vi "SERIAL_DecodeASCIIPacket.vi"(8 "error in":errorcluster, 9 "PacketType":string, 10 "Buffer":string, 11 "navX DevRef":T1={"SerialPortRef"={"DevStatus"={"status"=FALSE, "code"=0, "source"=""}, "Serial Port Name"=""}, "Board Information"={"WhoAmI (50 | 0x32)"=0, "Board Revision"=0, "Firmware Major Version"=0, "Firmware Minor Version"=0, "NAVX_BOARD_CAPABILITY"={"OMNIMOUNT"=FALSE, "YAW_RESET"=FALSE, "VEL_AND_DISP"=FALSE}, "NAVX_BOARD_YAW_AXIS"={"BOARD_YAW_AXIS_UP"=FALSE, "BOARD_YAW_AXIS"=0}}, "Status"={"Update Rate Hz"=0, "Accelerometer Full-Scale Range"=0, "Gyro Full-Scale Range"=0, "NAVX_OP_STATUS"=0, "NAVX_CAL_STATUS"=0, "NAVX_SELFTEST_STATUS"=0, "NAVX_SENSOR_STATUS"={"MOVING"=FALSE, "YAW_STABLE"=FALSE, "MAG_DISTURBANCE"=FALSE, "ALTITUDE_VALID"=FALSE, "SEALEVEL_PRESS_SET"=FALSE, "FUSED_HEADING_VALID"=FALSE}}, "Offsets"={"Yaw"=0.0, "Quat W"=0.0, "Quat X"=0.0, "Quat Y"=0.0, "Quat Z"=0.0}, "Update Rate (4Hz-60Hz)"=50, "Nav6Mode (YPR)"=enum."YPR", "refnum name"="", "error"={"status"=FALSE, "code"=0, "source"=""}, "Loop VI Refnum"=refnum, "Serial Port"=enum."Onboard RS-232"} {"Status"."NAVX_OP_STATUS" items=["INITIALIZING", "SELFTEST_IN_PROGRESS", "ERROR", "IMU_AUTOCAL_IN_PROGRESS", "NORMAL"]; "Status"."NAVX_CAL_STATUS" items=["IMU_CAL_STATE_MASK"=3, "IMU_CAL_INPROGRESS"=0, "IMU_CAL_ACCUMULATE"=1, "IMU_CAL_COMPLETE"=2, "MAG_CAL_COMPLETE"=4, "BARO_CAL_COMPLETE"=8]}) -> (0 "error out":errorcluster, 2 "Valid":bool, 3 "navX DevRef":T1={"SerialPortRef"={"DevStatus"={"status"=FALSE, "code"=0, "source"=""}, "Serial Port Name"=""}, "Board Information"={"WhoAmI (50 | 0x32)"=0, "Board Revision"=0, "Firmware Major Version"=0, "Firmware Minor Version"=0, "NAVX_BOARD_CAPABILITY"={"OMNIMOUNT"=FALSE, "YAW_RESET"=FALSE, "VEL_AND_DISP"=FALSE}, "NAVX_BOARD_YAW_AXIS"={"BOARD_YAW_AXIS_UP"=FALSE, "BOARD_YAW_AXIS"=0}}, "Status"={"Update Rate Hz"=0, "Accelerometer Full-Scale Range"=0, "Gyro Full-Scale Range"=0, "NAVX_OP_STATUS"=0, "NAVX_CAL_STATUS"=0, "NAVX_SELFTEST_STATUS"=0, "NAVX_SENSOR_STATUS"={"MOVING"=FALSE, "YAW_STABLE"=FALSE, "MAG_DISTURBANCE"=FALSE, "ALTITUDE_VALID"=FALSE, "SEALEVEL_PRESS_SET"=FALSE, "FUSED_HEADING_VALID"=FALSE}}, "Offsets"={"Yaw"=0.0, "Quat W"=0.0, "Quat X"=0.0, "Quat Y"=0.0, "Quat Z"=0.0}, "Update Rate (4Hz-60Hz)"=50, "Nav6Mode (YPR)"=enum."YPR", "refnum name"="", "error"={"status"=FALSE, "code"=0, "source"=""}, "Loop VI Refnum"=refnum, "Serial Port"=enum."Onboard RS-232"} {"Status"."NAVX_OP_STATUS" items=["INITIALIZING", "SELFTEST_IN_PROGRESS", "ERROR", "IMU_AUTOCAL_IN_PROGRESS", "NORMAL"]; "Status"."NAVX_CAL_STATUS" items=["IMU_CAL_STATE_MASK"=3, "IMU_CAL_INPROGRESS"=0, "IMU_CAL_ACCUMULATE"=1, "IMU_CAL_COMPLETE"=2, "MAG_CAL_COMPLETE"=4, "BARO_CAL_COMPLETE"=8]})   [LabVIEW 2014, in "navX-MXP IMU.lvlib"]
uses:
  navX-MXP IMU.lvlib
  navX Serial DevRef.ctl
  <vilib>/Rock Robotics/WPI/SerialPort/WPI_SerialPortRef.ctl
  COMMON/TypeDefs/Data TypeDefs/navX Board Information.ctl
  COMMON/TypeDefs/Value TypeDefs/navX NAVX_BOARD_CAPABILITY.ctl
  COMMON/TypeDefs/Value TypeDefs/navX NAVX_BOARD_YAW_AXIS.ctl
  COMMON/TypeDefs/Data TypeDefs/navX Status Data.ctl
  COMMON/TypeDefs/Value TypeDefs/navX NAVX_OP_STATUS.ctl
  COMMON/TypeDefs/Value TypeDefs/navX NAVX_CAL_STATUS.ctl
  COMMON/TypeDefs/Value TypeDefs/navX NAVX_SENSOR_STATUS.ctl
  TypeDefs/navX Serial Mode.ctl
  IO/NI WPI/WPI_SerialPort_USB.ctl
  COMMON/TypeDefs/Data TypeDefs/navX Vector Data.ctl
  TypeDefs/navX Raw Data.ctl
  COMMON/TypeDefs/Data TypeDefs/navX YPRH Data.ctl
  <vilib>/Rock Robotics/SystemInterfaces/Utilities/FPGA_UtilitiesRead LocalTime.vi
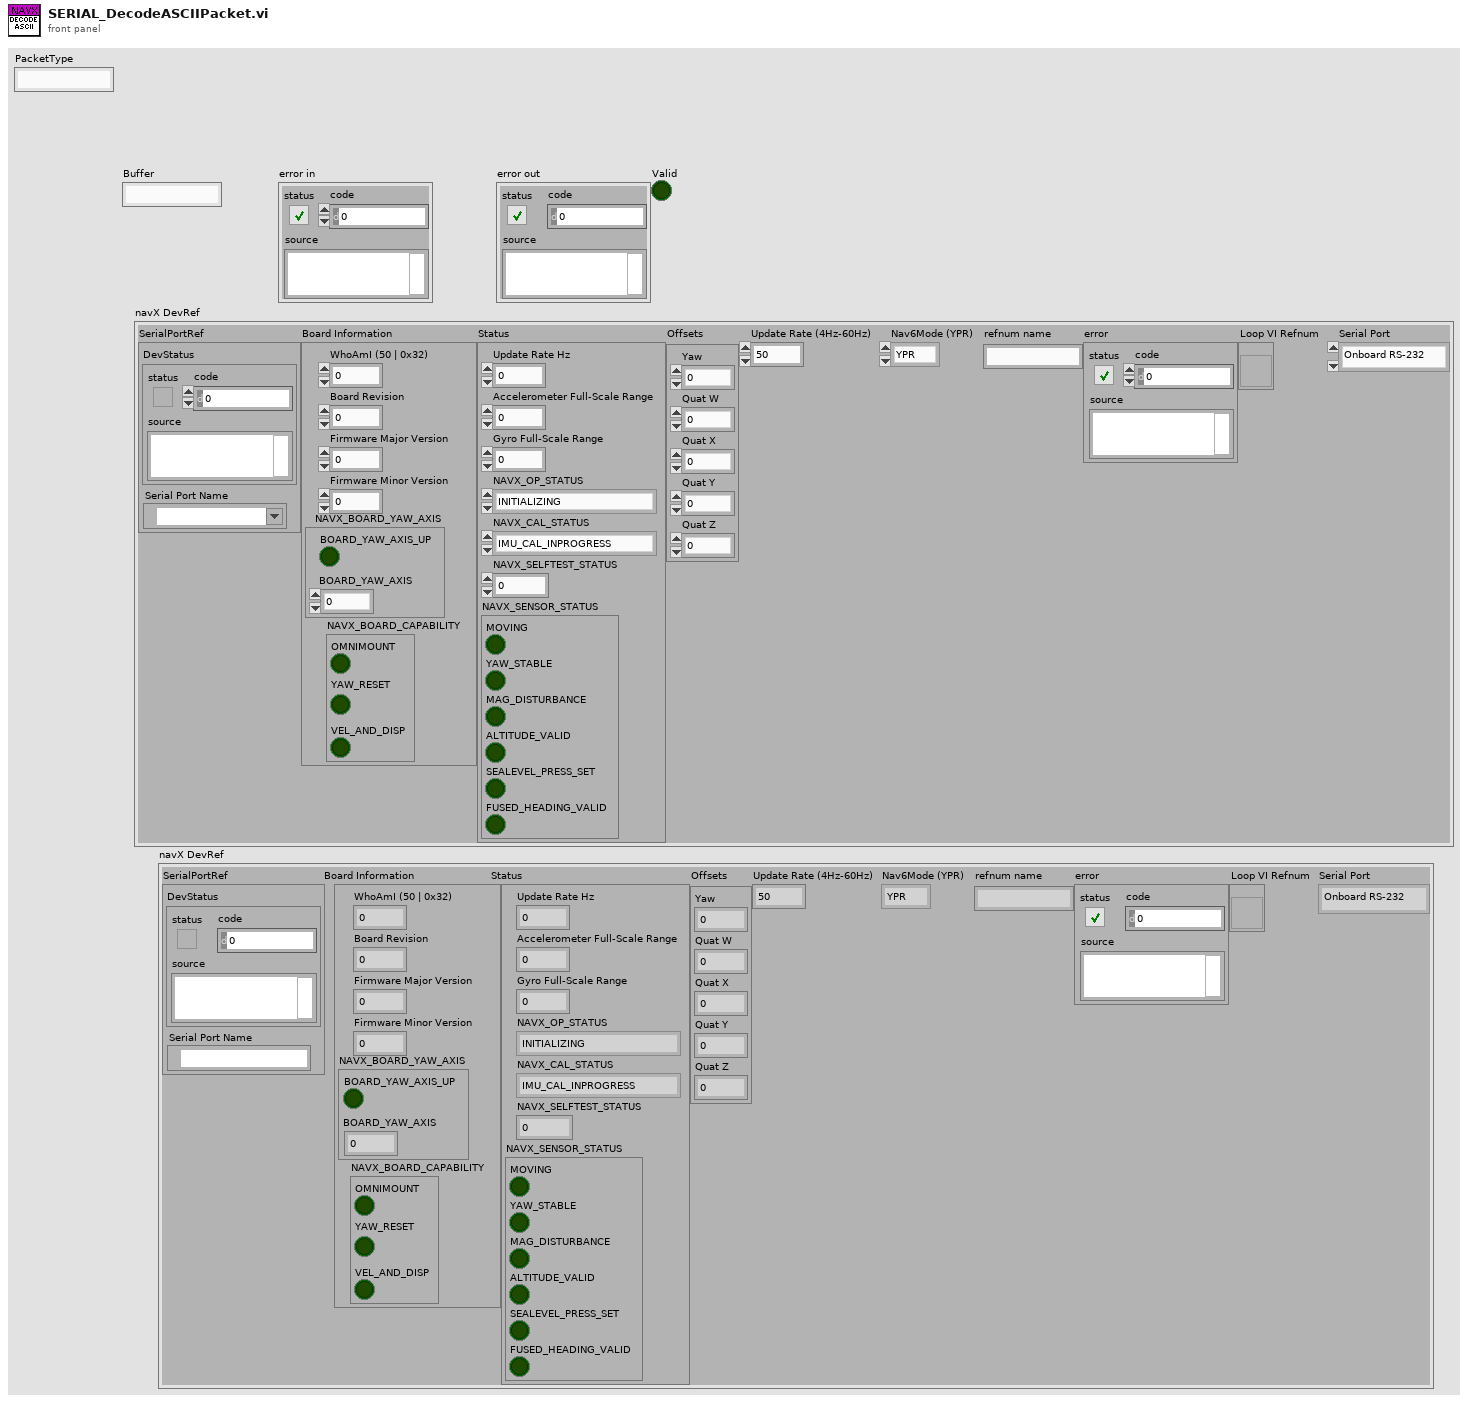
[diagram p1: front panel]
types:
  T1 = typedef "navX-MXP IMU.lvlib/navX Serial DevRef.ctl" = cluster{"SerialPortRef":T2, "Board Information":T3, "Status":T6, "Offsets":cluster{"Yaw":dbl, "Quat W":dbl, "Quat X":dbl, "Quat Y":dbl, "Quat Z":dbl}, "Update Rate (4Hz-60Hz)":u8, "Nav6Mode (YPR)":T10, "refnum name":string, "error":errorcluster, "Loop VI Refnum":refnum<vi>, "Serial Port":T11}
  T2 = typedef "WPI_SerialPortRef.ctl" = cluster{"DevStatus":errorcluster, "Serial Port Name":refnum<visa-resource-name>}
  T3 = typedef "navX-MXP IMU.lvlib/navX Board Information.ctl" = cluster{"WhoAmI (50 | 0x32)":u8, "Board Revision":u8, "Firmware Major Version":u8, "Firmware Minor Version":u8, "NAVX_BOARD_CAPABILITY":T4, "NAVX_BOARD_YAW_AXIS":T5}
  T4 = typedef "navX-MXP IMU.lvlib/navX NAVX_BOARD_CAPABILITY.ctl" = cluster{"OMNIMOUNT":bool, "YAW_RESET":bool, "VEL_AND_DISP":bool}
  T5 = typedef "navX-MXP IMU.lvlib/navX NAVX_BOARD_YAW_AXIS.ctl" = cluster{"BOARD_YAW_AXIS_UP":bool, "BOARD_YAW_AXIS":u8}
  T6 = typedef "navX-MXP IMU.lvlib/navX Status Data.ctl" = cluster{"Update Rate Hz":u8, "Accelerometer Full-Scale Range":u8, "Gyro Full-Scale Range":u16, "NAVX_OP_STATUS":T7, "NAVX_CAL_STATUS":T8, "NAVX_SELFTEST_STATUS":u8, "NAVX_SENSOR_STATUS":T9}
  T7 = typedef "navX-MXP IMU.lvlib/navX NAVX_OP_STATUS.ctl" = u8
  T8 = typedef "navX-MXP IMU.lvlib/navX NAVX_CAL_STATUS.ctl" = u8
  T9 = typedef "navX-MXP IMU.lvlib/navX NAVX_SENSOR_STATUS.ctl" = cluster{"MOVING":bool, "YAW_STABLE":bool, "MAG_DISTURBANCE":bool, "ALTITUDE_VALID":bool, "SEALEVEL_PRESS_SET":bool, "FUSED_HEADING_VALID":bool}
  T10 = typedef "navX-MXP IMU.lvlib/navX Serial Mode.ctl" = enum16{"YPR", "Gyro", "Quaternion", "AHRS", "AHRSPos"}
  T11 = typedef "navX-MXP IMU.lvlib/WPI_SerialPort_USB.ctl" = enum16{"Onboard RS-232", "MXP TTL", "USB"}
  T12 = cluster{"Gyroscope Full Scale Range":u32, "Accelerometer Full Scale Range":u32, "Update Rate":u32, "Calibrated Yaw Offset":dbl, "Calibrated Quaternion W Offset ":u32, "Calibrated Quaternion X Offset":u32, "Calibrated Quaternion Y Offset":u32, "Calibrated Quaternion Z Offset":u32, "Flags":u32}
  T13 = typedef "navX-MXP IMU.lvlib/navX Raw Data.ctl" = cluster{"RawAccel":T14, "RawGyro":T14, "RawMag":T14, "LastUpdateFPGATimestamp":dbl}
  T14 = typedef "navX-MXP IMU.lvlib/navX Vector Data.ctl" = cluster{"X":dbl, "Y":dbl, "Z":dbl}
  T15 = typedef "navX-MXP IMU.lvlib/navX YPRH Data.ctl" = cluster{"Yaw":dbl, "Pitch":dbl, "Roll":dbl, "Heading":dbl}
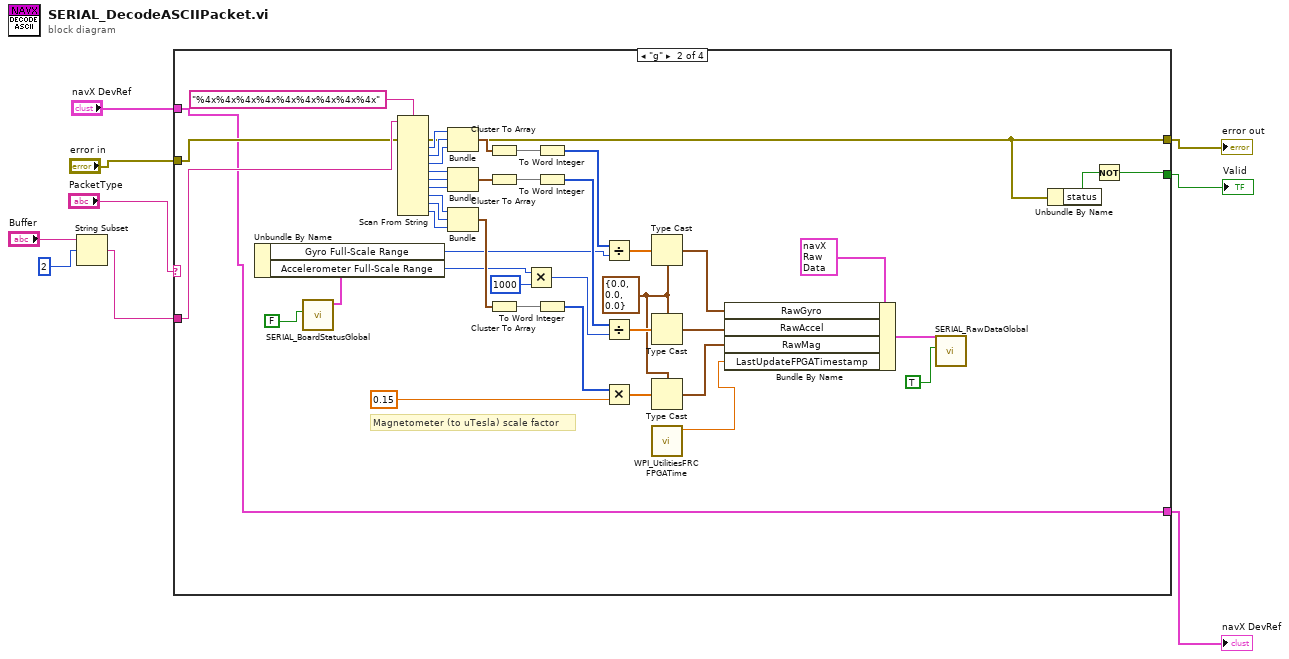
[diagram p0: block diagram]
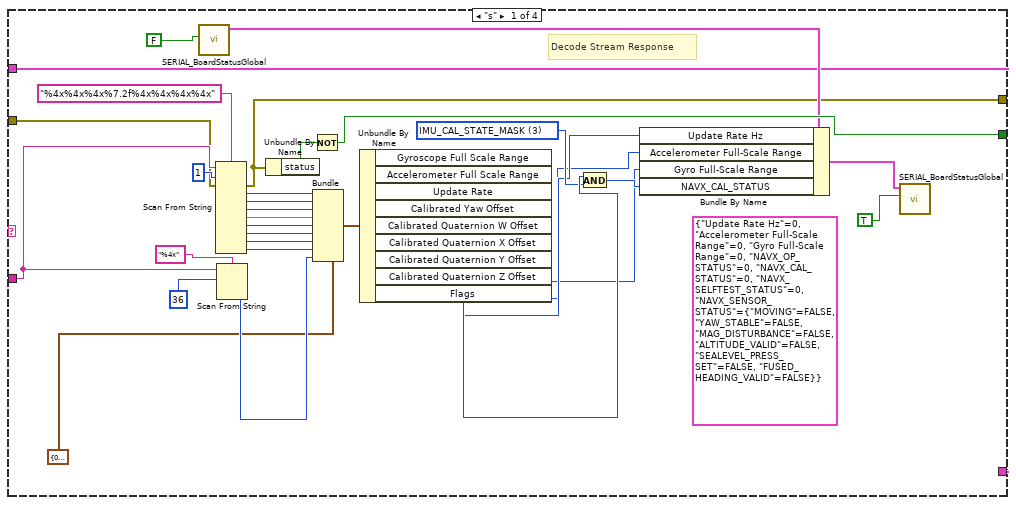
[diagram p2: hidden frame]
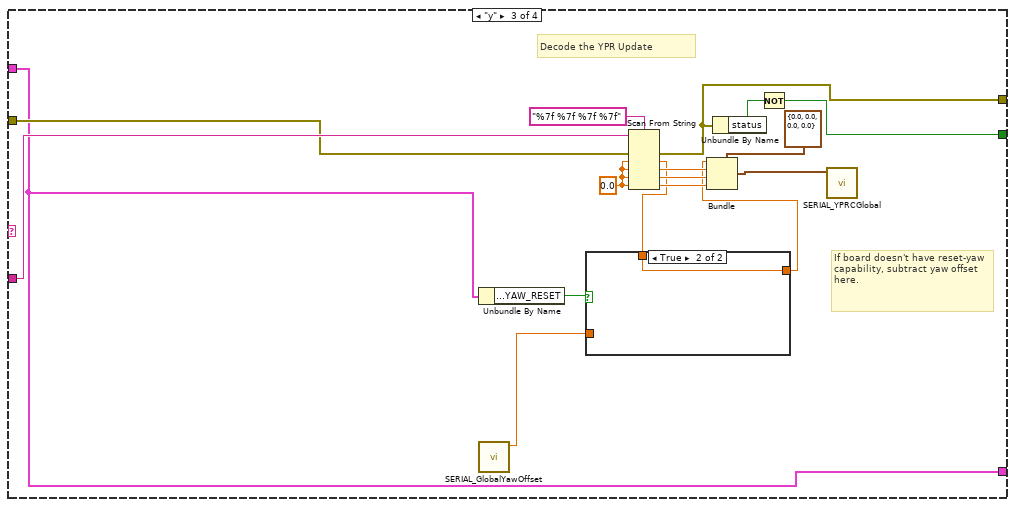
[diagram p3: hidden frame]
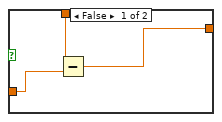
[diagram p4: hidden frame]
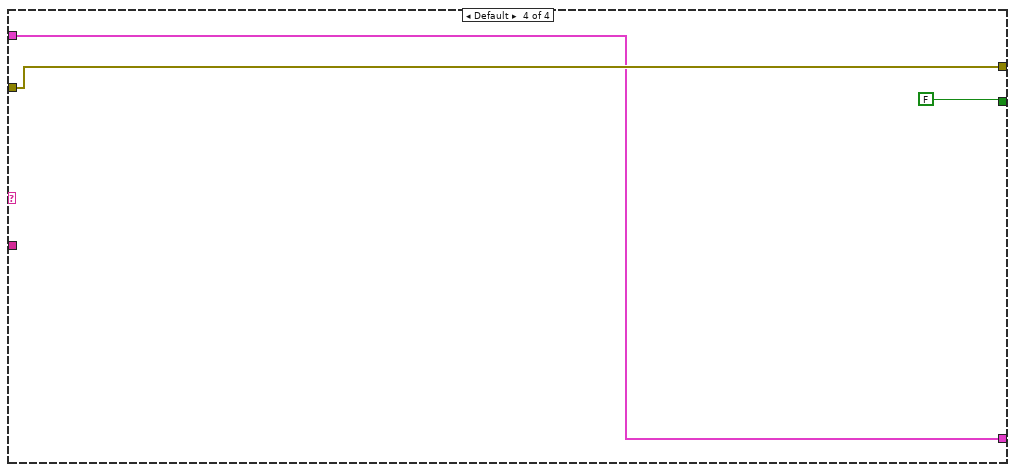
[diagram p5: hidden frame]
diagram:
  n1 = String Subset(string="Buffer", offset (0)=2) -> (substring=w3:string)  [unwired: 1 in]
  n2 = case shown="\"g\"" "PacketType" {
    tunnel: w3 -> [w31 w56 w94 _]
    tunnel: "error in" -> [w26 w55 w93 w106]
    tunnel: [w11 w45 w84 w105] -> w5
    tunnel: [w12 w53 w87 w106] -> w6
    tunnel: [w18 w52 w86 FALSE] -> w1
    tunnel: "navX DevRef" -> [w11 w45 w84 w105]
    frame "s" {
      (unwired) T6 {"Update Rate Hz"=0, "Accelerometer Full-Scale Range"=0, "Gyro Full-Scale Range"=0, "NAVX_OP_STATUS"=0, "NAVX_CAL_STATUS"=0, "NAVX_SELFTEST_STATUS"=0, "NAVX_SENSOR_STATUS"={"MOVING"=FALSE, "YAW_STABLE"=FALSE, "MAG_DISTURBANCE"=FALSE, "ALTITUDE_VALID"=FALSE, "SEALEVEL_PRESS_SET"=FALSE, "FUSED_HEADING_VALID"=FALSE}} ("Status")
      w23 = T8 3 items=["IMU_CAL_STATE_MASK"=3, "IMU_CAL_INPROGRESS"=0, "IMU_CAL_ACCUMULATE"=1, "IMU_CAL_COMPLETE"=2, "MAG_CAL_COMPLETE"=4, "BARO_CAL_COMPLETE"=8] ("NAVX_CAL_STATUS")
      # "Decode Stream Response"
      n3 = call "SERIAL_BoardStatusGlobal.vi"("Set"=FALSE) -> ("Status"=w14:T6)  [unwired: 9 in, 1 out]
      n4 = Scan From String(format string="%4x%4x%4x%7.2f%4x%4x%4x%4x", input string=w31, initial scan location=u32 1, error in=w26) -> (error out=w12:errorcluster, output 1=w33:u32, output 2=w34:u32, output 3=w35:u32, output 4=w40:dbl, output 5=w30:u32, output 6=w29:u32, output 7=w28:u32, output 8=w27:u32)  [unwired: 8 in, 2 out]
      n5 = Scan From String(format string="%4x", input string=w31, initial scan location=u32 36) -> (output 1=w39:u32)  [unwired: 2 in, 3 out]
      n6 = Unbundle By Name(w12) -> ("status"=w37:bool)
      n7 = Not(x=w37) -> (.not. x?=w18:bool)
      n8 = Bundle(cluster=T12 {"Gyroscope Full Scale Range"=0, "Accelerometer Full Scale Range"=0, "Update Rate"=0, "Calibrated Yaw Offset"=0.0, "Calibrated Quaternion W Offset "=0, "Calibrated Quaternion X Offset"=0, "Calibrated Quaternion Y Offset"=0, "Calibrated Quaternion Z Offset"=0, "Flags"=0}, "Gyroscope Full Scale Range"=w33, "Accelerometer Full Scale Range"=w34, "Update Rate"=w35, "Calibrated Yaw Offset"=w40, "Calibrated Quaternion W Offset"=w30, "Calibrated Quaternion X Offset"=w29, "Calibrated Quaternion Y Offset"=w28, "Calibrated Quaternion Z Offset"=w27, "Flags"=w39) -> (w19:T12)
      n9 = Unbundle By Name(w19) -> ("Gyroscope Full Scale Range"=w21:u32, "Accelerometer Full Scale Range"=w20:u32, "Update Rate"=w22:u32, "Flags"=w25:u32)  [unwired: 5 out]
      n10 = And(x=w25, y=w23) -> (x .and. y?=w24:u32)
      n11 = Bundle By Name(cluster=w14, "Update Rate Hz"=w22, "Accelerometer Full-Scale Range"=w20, "Gyro Full-Scale Range"=w21, "NAVX_CAL_STATUS"=w24) -> (w13:T6)
      n12 = call "SERIAL_BoardStatusGlobal.vi"("Set"=TRUE, "Status"=w13) -> ()  [unwired: 8 in, 2 out]
    }
    frame "g" {
      w59 = T14 {"X"=0.0, "Y"=0.0, "Z"=0.0} ("Vector")
      # "Magnetometer (to uTesla) scale factor"
      n13 = call "SERIAL_BoardStatusGlobal.vi"("Set"=FALSE) -> ("Status"=w43:T6)  [unwired: 9 in, 1 out]
      n14 = Unbundle By Name(w43) -> ("Gyro Full-Scale Range"=w42:u16, "Accelerometer Full-Scale Range"=w41:u8)
      n15 = Scan From String(format string="%4x%4x%4x%4x%4x%4x%4x%4x%4x", input string=w56, error in=w55) -> (error out=w53:errorcluster, output 1=w73:u32, output 2=w72:u32, output 3=w71:u32, output 4=w81:u32, output 5=w80:u32, output 6=w79:u32, output 7=w66:u32, output 8=w65:u32, output 9=w64:u32)  [unwired: 10 in, 2 out]
      n16 = Bundle(w73, w72, w71) -> (w69:cluster{u32, u32, u32})  [unwired: 1 in]
      n17 = Bundle(w81, w80, w79) -> (w78:cluster{u32, u32, u32})  [unwired: 1 in]
      n18 = Bundle(w66, w65, w64) -> (w62:cluster{u32, u32, u32})  [unwired: 1 in]
      n19 = Cluster To Array(cluster=w69) -> (array=w67:u32[])
      n20 = Cluster To Array(cluster=w78) -> (array=w77:u32[])
      n21 = Cluster To Array(cluster=w62) -> (array=w63:u32[])
      n22 = Multiply(x=w41, y=u16 1000) -> (x*y=w57:u16)
      n23 = To Word Integer(number=w67) -> (16bit integer=w70:i16[])
      n24 = To Word Integer(number=w77) -> (16bit integer=w76:i16[])
      n25 = To Word Integer(number=w63) -> (16bit integer=w61:i16[])
      n26 = Divide(x=w70, y=w42) -> (x/y=w68:dbl[])
      n27 = Divide(x=w76, y=w57) -> (x/y=w74:dbl[])
      n28 = Multiply(x=w61, y=0.15) -> (x*y=w58:dbl[])
      n29 = Type Cast(type=w59, x=w68) -> (*(type *) &x=w50:T14)
      n30 = Type Cast(type=w59, x=w74) -> (*(type *) &x=w49:T14)
      n31 = Type Cast(type=w59, x=w58) -> (*(type *) &x=w48:T14)
      n32 = call <vilib>:"WPI_UtilitiesFRC FPGATime.vi"() -> ("FPGA Time"=w47:dbl)  [unwired: 10 in, 1 out]
      n33 = Bundle By Name(cluster=T13 {"RawAccel"={"X"=0.0, "Y"=0.0, "Z"=0.0}, "RawGyro"={"X"=0.0, "Y"=0.0, "Z"=0.0}, "RawMag"={"X"=0.0, "Y"=0.0, "Z"=0.0}, "LastUpdateFPGATimestamp"=0.0} ("RawData"), "RawGyro"=w50, "RawAccel"=w49, "RawMag"=w48, "LastUpdateFPGATimestamp"=w47) -> (w46:T13)
      n34 = call "SERIAL_RawDataGlobal.vi"("Set"=TRUE, "RawData"=w46) -> ()  [unwired: 9 in, 1 out]
      n35 = Unbundle By Name(w53) -> ("status"=w54:bool)
      n36 = Not(x=w54) -> (.not. x?=w52:bool)
    }
    frame "y" {
      w100 = 0.0 ("default value 4")
      # "If board doesn't have reset-yaw capability, subtract yaw offset here."
      # "Decode the YPR Update"
      n37 = Unbundle By Name(w84) -> ("Board Information.NAVX_BOARD_CAPABILITY.YAW_RESET"=w92:bool)
      n38 = call "SERIAL_GlobalYawOffset.vi"() -> ("OutputYawOffset"=w85:dbl)  [unwired: 11 in]
      n39 = Scan From String(format string="%7f %7f %7f %7f", input string=w94, error in=w93, default 1=w100, default 2=w100, default 3=w100, default 4=w100) -> (error out=w87:errorcluster, output 1=w91:dbl, output 2=w97:dbl, output 3=w98:dbl, output 4=w99:dbl)  [unwired: 1 in, 2 out]
      n40 = case shown="True" w92 {
        tunnel: w85 -> [w103 _]
        tunnel: w91 -> [w102 w104]
        tunnel: [w101 w104] -> w90
        frame False {
          n41 = Subtract(x=w102, y=w103) -> (x-y=w101:dbl)
        }
        frame True {
        }
      }
      n42 = Bundle(cluster=T15 {"Yaw"=0.0, "Pitch"=0.0, "Roll"=0.0, "Heading"=0.0} ("YPR Update"), "Yaw"=w90, "Pitch"=w97, "Roll"=w98, "Heading"=w99) -> (w89:T15)
      n43 = Unbundle By Name(w87) -> ("status"=w88:bool)
      n44 = Not(x=w88) -> (.not. x?=w86:bool)
      n45 = call "SERIAL_YPRCGlobal.vi"("YPRH"=w89) -> ()  [unwired: 9 in, 2 out]
    }
    frame Default {
    }
  }
  "error out" <- w6
  "Valid" <- w1
  "navX DevRef" <- w5
